vi "KE6221 -- Set Wave Amplitude tmp.vi"(0 "Resource In":refnum<visa-resource-name>, 1 "Check For SCPI Errors? (T)":bool=TRUE, 7 "Wave Amplitude In":T1=0.001 min=2e-12 max=0.105 format="%.3p", 11 "error in (no error)":errorcluster, 12 "Read Back Set Value? (T)":bool=TRUE) -> (4 "Resource Out (dupl)":refnum<visa-resource-name>, 8 "Wave Amplitude Out":T1=0.001 min=2e-12 max=0.105 format="%.3p", 15 "error out":errorcluster)   [LabVIEW 2015, in "Keithley 622x tmp.lvlib"]
uses:
  Keithley 622x tmp.lvlib
  Typedefs/KE6221 -- Wave Amplitude tmp.ctl
panel:
  out "String":string
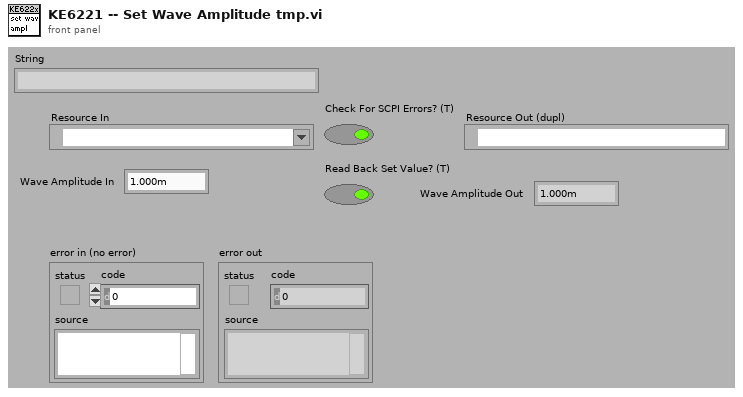
[diagram p1: front panel]
types:
  T1 = typedef "Keithley 622x tmp.lvlib/KE6221 -- Wave Amplitude tmp.ctl" = dbl
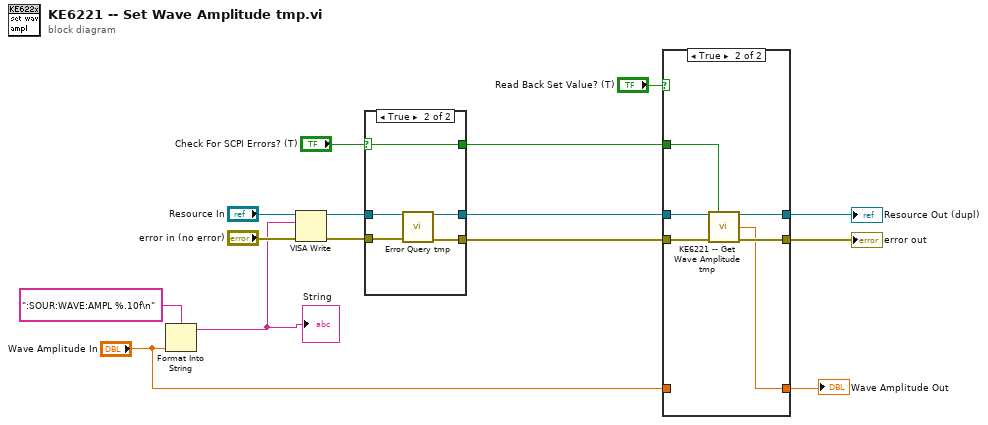
[diagram p0: block diagram]
diagram:
  n1 = Format Into String(format string=":SOUR:WAVE:AMPL %.10f\n", "Wave Amplitude In") -> (resulting string=w1:string)  [unwired: 2 in, 1 out]
  "String" <- w1
  n2 = VISA Write(VISA resource name="Resource In", write buffer=w1, error in (no error)="error in (no error)") -> (VISA resource name out=w11:refnum<visa-resource-name>, error out=w10:errorcluster)  [unwired: 1 out]
  n3 = case shown="True" "Check For SCPI Errors? (T)" {
    selector: "Check For SCPI Errors? (T)" -> [w16 w19]
    tunnel: w11 -> [w18 w23]
    tunnel: w10 -> [w17 w22]
    tunnel: [w17 w21] -> w6
    tunnel: [w18 w20] -> w9
    tunnel: [w16 w19] -> w7
    frame False {
    }
    frame True {
      n4 = call "Error Query tmp.vi"("VISA Resource In"=w23, "error in (no error)"=w22) -> ("VISA Resource Out (dupl)"=w20:refnum<visa-resource-name>, "error out"=w21:errorcluster)  [unwired: 10 in, 2 out]
    }
  }
  n5 = case shown="True" "Read Back Set Value? (T)" {
    tunnel: w9 -> [w25 w32]
    tunnel: w7 -> [_ w31]
    tunnel: w6 -> [w24 w30]
    tunnel: "Wave Amplitude In" -> [w26 _]
    tunnel: [w26 w27] -> w2
    tunnel: [w25 w29] -> w5
    tunnel: [w24 w28] -> w4
    frame False {
    }
    frame True {
      n6 = call "KE6221 -- Get Wave Amplitude tmp.vi"("Resource In"=w32, "Check For SCPI Errors? (T)"=w31, "error in (no error)"=w30) -> ("Resource Out (dupl)"=w29:refnum<visa-resource-name>, "Wave Amplitude"=w27:T1, "error out"=w28:errorcluster)  [unwired: 10 in]
    }
  }
  "Resource Out (dupl)" <- w5
  "error out" <- w4
  "Wave Amplitude Out" <- w2
